vi "EXA_logEvent_RejectedCommand.vi"(8 "error in (no error)":errorcluster, 11 "logevent_RejectedCommand_Ctl":T1) -> (0 "error out":errorcluster, 2 "function return":i32, 3 "logevent_RejectedCommand_Ctl out":T1)   [LabVIEW 2016, in "SALLV_EXA.lvlib"]
doc: "int EXA_shm_logEvent_RejectedCommandLV(EXA_logevent_RejectedCommandLV *logevent_RejectedCommand_Ctl );"
uses:
  SALLV_EXA.lvlib
  DataTypes/logevent_RejectedCommand.ctl
  SALLV_EXA.so
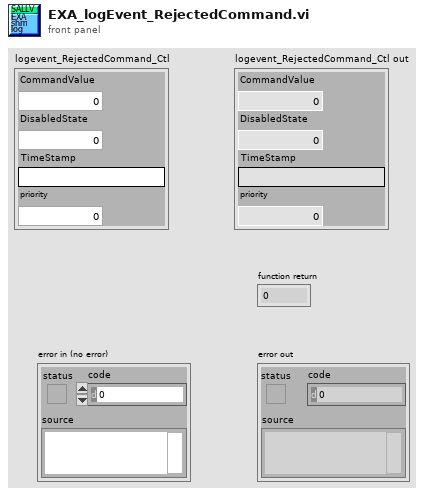
[diagram p1: front panel]
types:
  T1 = typedef "SALLV_EXA.lvlib/logevent_RejectedCommand.ctl" = cluster{"CommandValue":u16, "DisabledState":u16, "TimeStamp":string, "priority":i32}
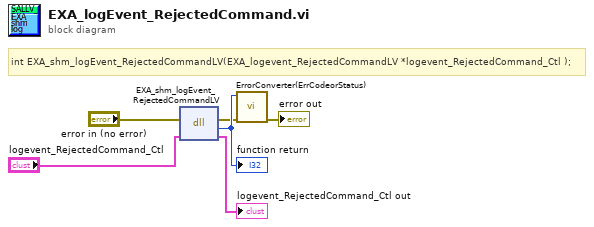
[diagram p0: block diagram]
diagram:
  # "int EXA_shm_logEvent_RejectedCommandLV(EXA_logevent_RejectedCommandLV *logevent_RejectedCommand_Ctl );"
  n1 = dll-call lib="home/andres/Desktop/EXA_SAL_LV/SALLV_EXA.*" fn="EXA_shm_logEvent_RejectedCommandLV"(error in="error in (no error)", "logevent_RejectedCommand_Ctl"="logevent_RejectedCommand_Ctl") -> (error out=w2:errorcluster, w6:i32, "logevent_RejectedCommand_Ctl"=→"logevent_RejectedCommand_Ctl out":T1)  [unwired: 2 in, 1 out]
  "function return" <- w6
  n2 = call "ErrorConverter(ErrCodeorStatus).vi"("error in (no error)"=w2, "error code"=w6) -> ("error out"=→"error out":errorcluster)  [unwired: 9 in]
